vi "Manufacturing-LoadAllSteps.vi"(8 "error in (no error)":errorcluster, 11 "ERP-CreateInstructions in":refnum<class "ERP-CreateInstructions.lvclass">) -> (0 "error out":errorcluster, 2 "All Part# Info":T1(array[cluster]), 3 "ERP-CreateInstructions out":refnum<class "ERP-CreateInstructions.lvclass">, 5 "Part Number":string)   [LabVIEW 2013, in "ERP-CreateInstructions.lvclass"]
uses:
  ERP-CreateInstructions.lvclass
  ERP-CreateInstructions.lvclass/ERP-CreateInstructions.ctl
  <userlib>/_OpenG.lib/string/string.llb/Trim Whitespace (String Array)__ogtk.vi
  <userlib>/_OpenG.lib/array/array.llb/Search 1D Array (String)__ogtk.vi
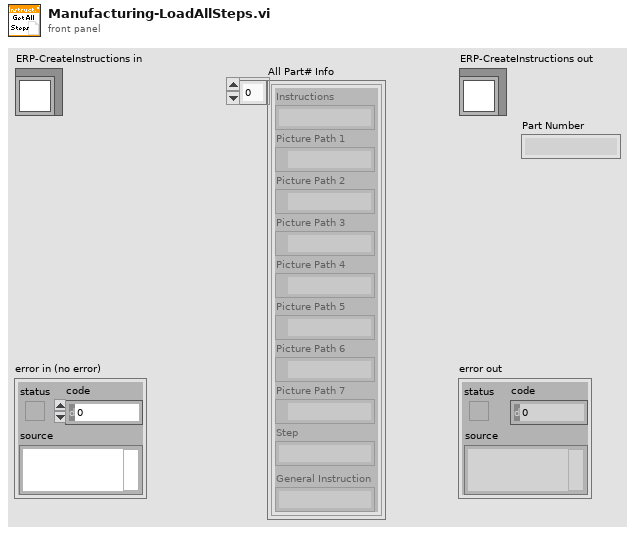
[diagram p1: front panel]
types:
  T1 = cluster{"Instructions":string, "Picture Path 1":path, "Picture Path 2":path, "Picture Path 3":path, "Picture Path 4":path, "Picture Path 5":path, "Picture Path 6":path, "Picture Path 7":path, "Step":string, "General Instruction":string}[]
  T2 = cluster{"Instructions":string, "Picture Path 1":path, "Picture Path 2":path, "Picture Path 3":path, "Picture Path 4":path, "Picture Path 5":path, "Picture Path 6":path, "Picture Path 7":path, "Step":string, "General Instruction":string}
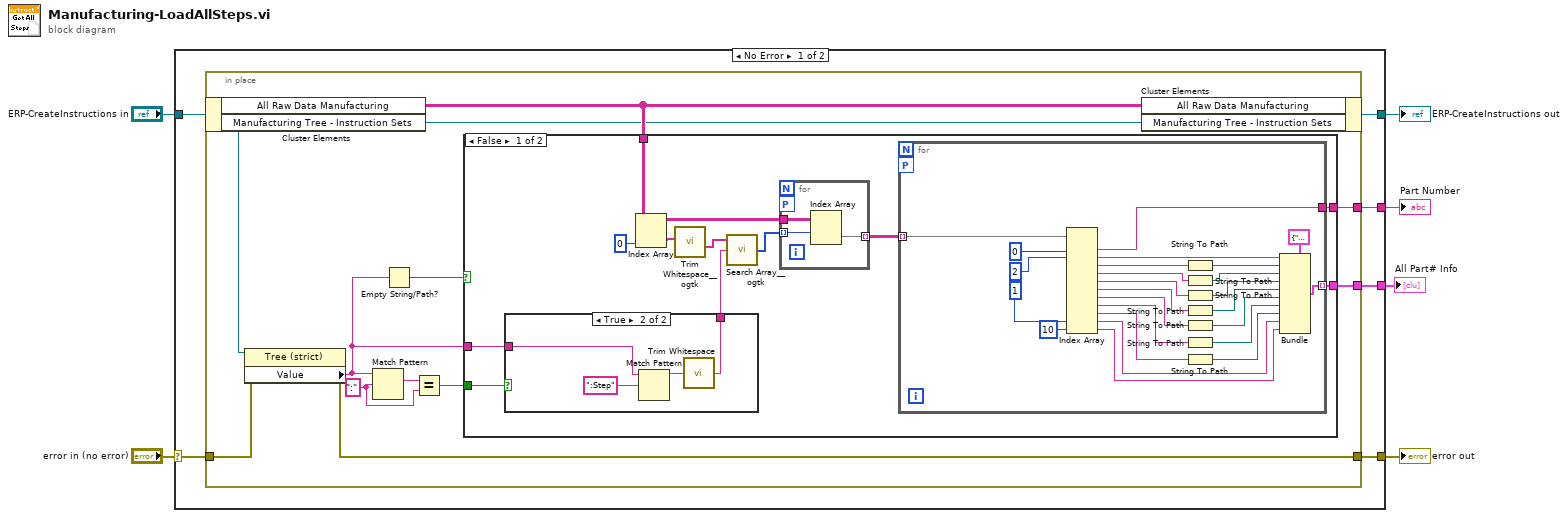
[diagram p0: block diagram]
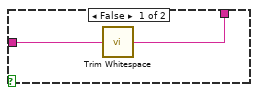
[diagram p2: hidden frame]
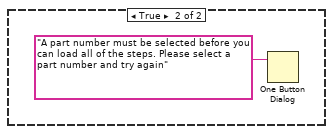
[diagram p3: hidden frame]
diagram:
  n1 = case shown="No Error" "error in (no error)" {
    selector: "error in (no error)" -> [w12 w71]
    tunnel: [w9 w71] -> w5
    tunnel: [w7 w70] -> w3
    tunnel: "ERP-CreateInstructions in" -> [w8 w70]
    tunnel: [w11 _] -> w2
    tunnel: [w10 _] -> w1
    frame No Error {
      n2 = in-place {
        in-place-border: w12 -> [w23]
        in-place-border: [w19] -> w10
        in-place-border: [w20] -> w9
        in-place-border: [w18] -> w11
        w15 = ":" ("regular expression")
        n3 = in-place-cluster #1(w8) -> ("All Raw Data Manufacturing"=w22:string[][], "Manufacturing Tree - Instruction Sets"=w21:refnum<vi>)
        n4 = property class="Tree (strict)"(reference=w21, error in=w23) -> (error out=w20:errorcluster, "Value"=w13:string)  [unwired: 1 out]
        n5 = Match Pattern(string=w13, regular expression=w15) -> (match substring=w16:string)  [unwired: 1 in, 3 out]
        n6 = Empty String/Path?(string/path=w13) -> (empty?=w17:bool)
        n7 = Equal?(x=w16, y=w15) -> (x = y?=w14:bool)
        n8 = case shown="False" w17 {
          tunnel: w22 -> [w31 _]
          tunnel: [w30 _] -> w19
          tunnel: [w29 _] -> w18
          tunnel: w14 -> [w25 _]
          tunnel: w13 -> [w24 _]
          frame False {
            n9 = case shown="True" w25 {
              tunnel: [w35 w38] -> w33
              tunnel: w24 -> [w36 w37]
              frame False {
                n10 = call <vilib>:"Trim Whitespace.vi"("string"=w36) -> ("trimmed string"=w35:string)  [unwired: 1 in]
              }
              frame True {
                n11 = Match Pattern(string=w37, regular expression=":Step") -> (before substring=w39:string)  [unwired: 1 in, 3 out]
                n12 = call <vilib>:"Trim Whitespace.vi"("string"=w39) -> ("trimmed string"=w38:string)  [unwired: 1 in]
              }
            }
            n13 = Index Array(array=w31, index (col)=0 ("disabled index (col)")) -> (element=w28:string[])  [unwired: 1 in]
            n14 = call-poly <userlib>:"Trim Whitespace__ogtk.vi"("String in"=w28) -> ("String out"=w27:string[])  [unwired: 6 in]
            n15 = call-poly <userlib>:"Search Array__ogtk.vi"("Array"=w27, "Element Data"=w33) -> ("Indices of Elements"=w32:i32[])  [unwired: 7 in]
            n16 = for {
              tunnel: w31 -> [w68]
              tunnel: w32 -> [w67] mode=indexing
              tunnel: [w66] -> w26 mode=indexing
              workers-P: _ -> [_]
              n17 = Index Array(array=w68, index (row)=w67) -> (element=w66:string[])  [unwired: 1 in]
            }
            n18 = for {
              tunnel: [w58] -> w30 mode=indexing
              tunnel: [w55] -> w29
              tunnel: w26 -> [w43] mode=indexing
              workers-P: _ -> [_]
              n19 = Index Array(array=w43, index #1=0 ("index"), index #2=2 ("index"), index #10=1 ("index"), index #11=10 ("index")) -> (element #1=w55:string, element #2=w57:string, element #3=w65:string, element #4=w64:string, element #5=w63:string, element #6=w62:string, element #7=w61:string, element #8=w60:string, element #9=w59:string, element #10=w44:string, element #11=w41:string)  [unwired: 7 in]
              n20 = String To Path(string=w65) -> (path=w56:path)
              n21 = String To Path(string=w64) -> (path=w54:path)
              n22 = String To Path(string=w63) -> (path=w53:path)
              n23 = String To Path(string=w62) -> (path=w52:path)
              n24 = String To Path(string=w61) -> (path=w51:path)
              n25 = String To Path(string=w60) -> (path=w50:path)
              n26 = String To Path(string=w59) -> (path=w49:path)
              n27 = Bundle(cluster=T2 {"Instructions"="", "Picture Path 1"=path "", "Picture Path 2"=path "", "Picture Path 3"=path "", "Picture Path 4"=path "", "Picture Path 5"=path "", "Picture Path 6"=path "", "Picture Path 7"=path "", "Step"="", "General Instruction"=""}, "Instructions"=w57, "Picture Path 1"=w56, "Picture Path 2"=w54, "Picture Path 3"=w53, "Picture Path 4"=w52, "Picture Path 5"=w51, "Picture Path 6"=w50, "Picture Path 7"=w49, "Step"=w44, "General Instruction"=w41) -> (w58:T2)
            }
          }
          frame True {
            n28 = One Button Dialog(message="A part number must be selected before you can load all of the steps. Please select a part number and try again") -> ()  [unwired: 1 in, 1 out]
          }
        }
        n29 = in-place-cluster #1("All Raw Data Manufacturing"=w22, "Manufacturing Tree - Instruction Sets"=w21) -> (w7:refnum<class "ERP-CreateInstructions.lvclass">)
      }
    }
    frame Error {
    }
  }
  "error out" <- w5
  "ERP-CreateInstructions out" <- w3
  "Part Number" <- w2
  "All Part# Info" <- w1
